vi "update-experiments-group-listSD.vi"(0 "Experiments groups":refnum<class "Experiments_group.lvclass">[](array[class]), 2 "Group":refnum<vi>, 3 "error in (no error)":errorcluster) -> (9 "error out":errorcluster)   [LabVIEW 2015]
uses:
  Classes/Experiments/Experiments_group.lvclass
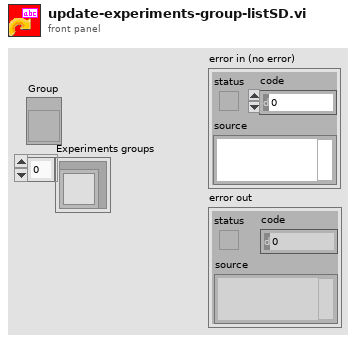
[diagram p1: front panel]
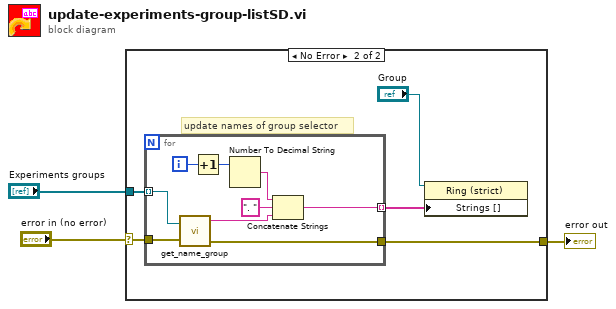
[diagram p0: block diagram]
diagram:
  n1 = case shown="No Error" "error in (no error)" {
    selector: "error in (no error)" -> [w4 w6]
    tunnel: "Experiments groups" -> [_ w7]
    tunnel: [w4 w5] -> w1
    frame Error {
    }
    frame No Error {
      # "update names of group selector"
      n2 = for {
        tunnel: w7 -> [w13] mode=indexing
        tunnel: [w16] -> w9 mode=indexing
        tunnel: w6 -> [w10]
        tunnel: [w11] -> w5
        i -> [w18]
        n3 = call-dynamic "get_name_group.vi"("Experiments_group.lvclass in"=w13, "error in (no error)"=w10) -> ("Name"=w12:string, "error out"=w11:errorcluster)  [unwired: 1 out]
        n4 = Increment(x=w18) -> (x+1=w15:i32)
        n5 = Number To Decimal String(number=w15) -> (decimal integer string=w14:string)  [unwired: 1 in]
        n6 = Concatenate Strings(w14, ". " ("string"), w12) -> (w16:string)
      }
      n7 = property on="Property Node" class="Ring (strict)"(reference="Group", "Strings []"=w9) -> ()  [unwired: 1 in, 2 out]
    }
  }
  "error out" <- w1
